vi "ge_AntiPDFlicker.vi"(5 "CellSize":T1) -> (2 "CellSize":T1)   [LabVIEW 2012]
uses:
  <vilib>/Utility/miscctls.llb/LVBoundsTypeDef.ctl
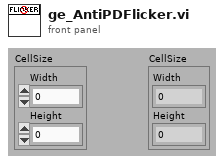
[diagram p1: front panel]
types:
  T1 = typedef "LVBoundsTypeDef.ctl" = cluster{"Width":u32, "Height":u32}
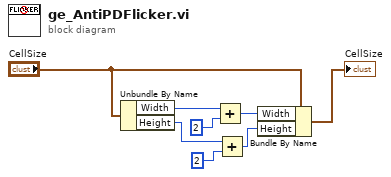
[diagram p0: block diagram]
diagram:
  n1 = Unbundle By Name("CellSize") -> ("Width"=w1:u32, "Height"=w7:u32)
  n2 = Add(x=w1, y=u32 2) -> (x+y=w2:u32)
  n3 = Add(x=w7, y=u32 2) -> (x+y=w8:u32)
  n4 = Bundle By Name(cluster="CellSize", "Width"=w2, "Height"=w8) -> (→"CellSize":T1)
